vi "re_LuaVIEW Cleanup Tasks.vi"   [LabVIEW 2012]
doc: "This VI is run by the registery daemon on receiving an application exit event. It attempts to clean up any remaining tasks by sending stop and confirm signals and, if applicable, changing to the \"stop\" runlevel of a running server.\n\nThis VI is statically linked into the \"Prepare Task\" VI so that it is only loaded when the task infrastructure is being used. It is run by the registery daemon only when loaded. This prevents the task infrastructure from being loaded when not in use."
uses:
  typedefs/t_LuaVIEW Task List Methods.ctl
types:
  T1 = typedef "t_LuaVIEW Task List Methods.ctl" = enum16{"clear list", "add", "test", "remove", "get ref", "get task info", "get list", "get script info", "ongoing?", "resume", "pause", "stop", "confirm", "message"}
  T2 = typedef "LuaVIEW Task Info.ctl" = cluster{"main script":string, "identifier":string, "class":string, "description":string, "mode":T3, "handler":string, "LuaVIEW reference":T4, "scripts":i32, "hide":bool, "active":bool, "error msg":string, "defer":bool, "launch":enum16{"asynchronous", "manual", "synchronous"}, "main path valid":bool, "start time":dbl, "swap time":dbl, "task VI":refnum<vi>, "prefsys":enum32{"invalid execution system", "user interface", "standard", "instrument i/o", "data acquisition", "other 1", "other 2", "same as caller"}, "priority":enum32{"invalid priority", "background priority", "normal priority", "above normal priority", "high priority", "time critical priority", "subroutine"}, "signal flags":u32, "allow mask":u32, "handle mask":u32, "disallow manual":bool}
  T3 = typedef "t_LuaVIEW Task Modes.ctl" = enum16{"initializing", "running", "executing", "paused", "error", "swapping"}
  T4 = typedef "t_LuaVIEW Reference.ctl" = refnum<k1>
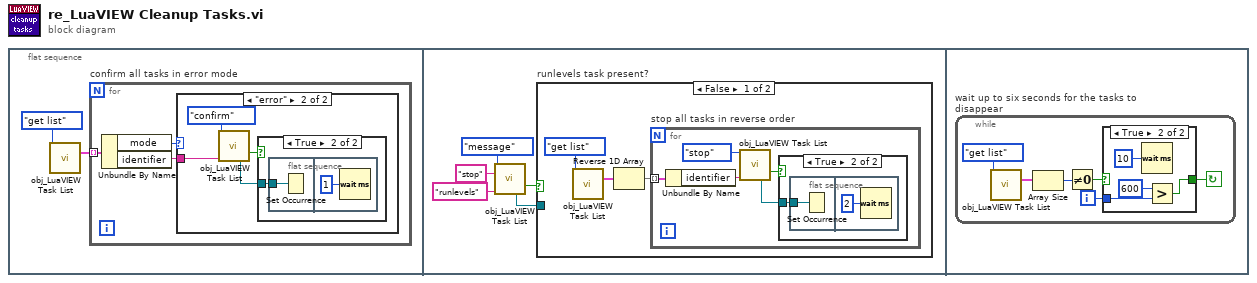
[diagram p0: block diagram]
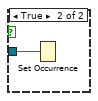
[diagram p5: hidden frame]
diagram:
  n1 = flat-sequence {
    frame #0 {
      n2 = call "obj_LuaVIEW Task List.vi"("method"=t_LuaVIEW_Task_List_Methods."get list") -> ("task info list"=w1:T2[])  [unwired: 9 in, 5 out]
      n3 = for "confirm all tasks in error mode" {
        tunnel: w1 -> [w5] mode=indexing
        n4 = Unbundle By Name(w5) -> ("mode"=w4:T3, "identifier"=w3:string)
        n5 = case shown="\"error\"" w4 {
          tunnel: w3 -> [_ w8]
          frame Default {
          }
          frame "error" {
            n6 = call "obj_LuaVIEW Task List.vi"("method"=t_LuaVIEW_Task_List_Methods."confirm", "task identifier"=w8) -> ("set/ongoing"=w7:bool, "wakeup occurrence"=w6:refnum<k4>)  [unwired: 8 in, 4 out]
            n7 = case shown="True" w7 {
              tunnel: w6 -> [_ w10]
              frame False {
              }
              frame True {
                n8 = flat-sequence {
                  tunnel: w10 -> [w11]
                  frame #0 {
                    n9 = Set Occurrence(w11) -> ()
                  }
                  frame #1 {
                    n10 = Wait (ms)(milliseconds to wait=u32 1) -> ()  [unwired: 1 out]
                  }
                }
              }
            }
          }
        }
      }
    }
    frame #1 {
      n11 = call "obj_LuaVIEW Task List.vi"("method"=t_LuaVIEW_Task_List_Methods."message", "message"="stop", "task identifier"="runlevels") -> ("set/ongoing"=w14:bool, "wakeup occurrence"=w13:refnum<k4>)  [unwired: 7 in, 4 out]
      n12 = case "runlevels task present?" shown="False" w14 {
        tunnel: w13 -> [_ w29]
        frame False {
          n13 = call "obj_LuaVIEW Task List.vi"("method"=t_LuaVIEW_Task_List_Methods."get list") -> ("task info list"=w20:T2[])  [unwired: 9 in, 5 out]
          n14 = Reverse 1D Array(array=w20) -> (reversed array=w18:T2[])
          n15 = for "stop all tasks in reverse order" {
            tunnel: w18 -> [w25] mode=indexing
            n16 = Unbundle By Name(w25) -> ("identifier"=w23:string)
            n17 = call "obj_LuaVIEW Task List.vi"("method"=t_LuaVIEW_Task_List_Methods."stop", "task identifier"=w23) -> ("set/ongoing"=w22:bool, "wakeup occurrence"=w21:refnum<k4>)  [unwired: 8 in, 4 out]
            n18 = case shown="True" w22 {
              tunnel: w21 -> [_ w26]
              frame False {
              }
              frame True {
                n19 = flat-sequence {
                  tunnel: w26 -> [w27]
                  frame #0 {
                    n20 = Set Occurrence(w27) -> ()
                  }
                  frame #1 {
                    n21 = Wait (ms)(milliseconds to wait=u32 2) -> ()  [unwired: 1 out]
                  }
                }
              }
            }
          }
        }
        frame True {
          n22 = Set Occurrence(w29) -> ()
        }
      }
    }
    frame #2 {
      n23 = while "wait up to six seconds for the tasks to disappear" {
        i -> [w30]
        stop <- w31 continue-if-true
        n24 = call "obj_LuaVIEW Task List.vi"("method"=t_LuaVIEW_Task_List_Methods."get list") -> ("task info list"=w34:T2[])  [unwired: 9 in, 5 out]
        n25 = Array Size(array=w34) -> (size(s)=w33:i32)
        n26 = Not Equal To 0?(x=w33) -> (x != 0?=w32:bool)
        n27 = case shown="True" w32 {
          selector: w32 -> [w36 _]
          tunnel: [w36 w37] -> w31
          tunnel: w30 -> [_ w39]
          frame False {
          }
          frame True {
            n28 = Wait (ms)(milliseconds to wait=u32 10) -> ()  [unwired: 1 out]
            n29 = Greater?(x=600, y=w39) -> (0:w37:bool)
          }
        }
      }
    }
  }
